vi "Show Animated Busy Icon with Message and Abort Button.vi"(2 "Already active? (F)":bool, 3 "Message":string, 7 "Target VI reference":refnum<vi>, 11 "Error In":errorcluster, 16 "Abort Button Name (Abort)":string="Abort", 17 "Animated Busy Icon Control Name (Animated Busy Icon)":string="Animated Busy Icon", 18 "Message Control Name (Message)":string="Message") -> (10 "Error Out":errorcluster)   [LabVIEW 2021, in "GUI.lvlib"]
doc: "This VI uses error in normally (doesn't do anything if there is an error in) and passes through the error in (ignores additional unternal errors)."
uses:
  GUI/GUI.lvlib
  Utilities/Utilities.lvlib
  Error/Error.lvlib
panel:
  # "see the License on the block diagram (Ctrl+E or Window:Show Block Diagram)"
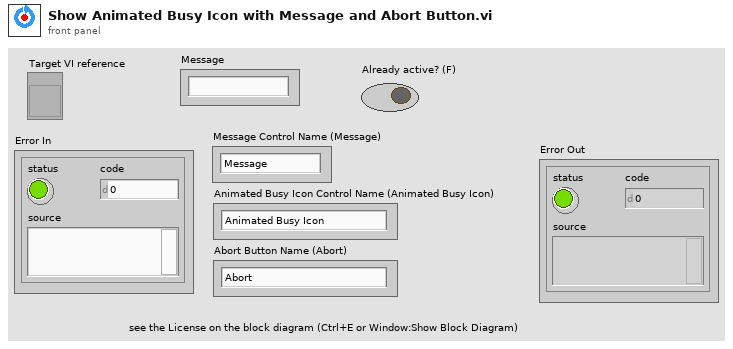
[diagram p1: front panel]
types:
  T1 = enum16{"Controls & Indicators", "Controls", "Indicators"}
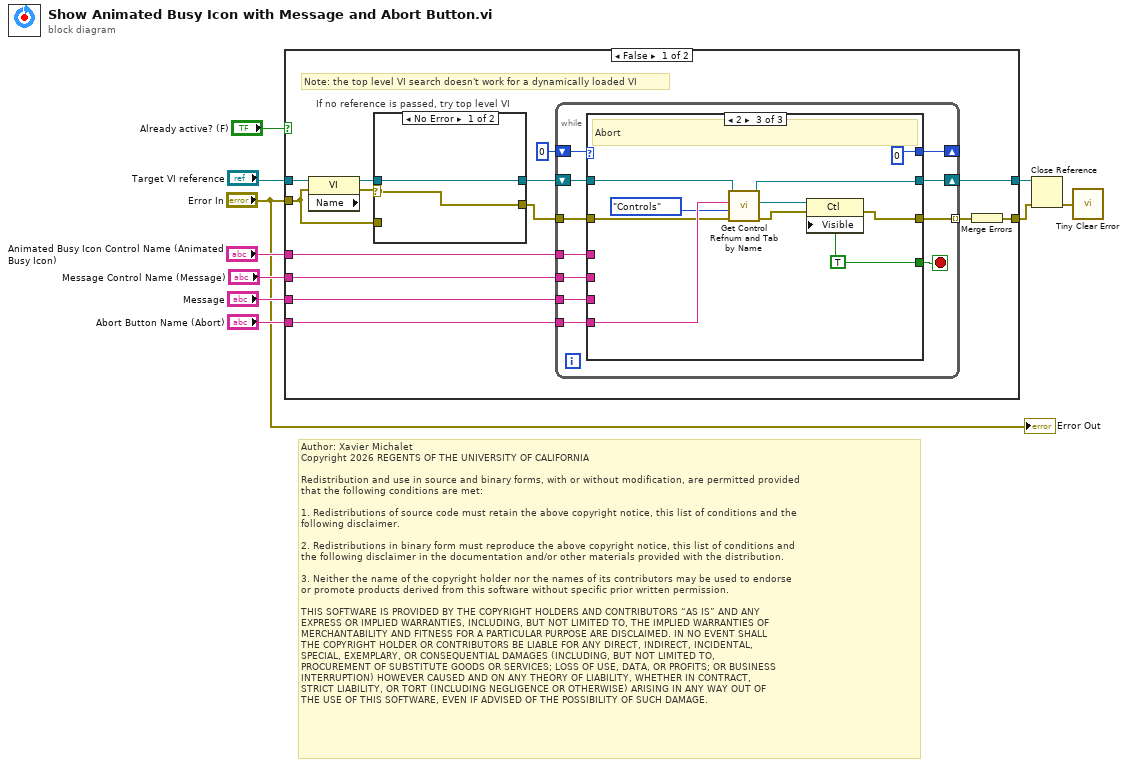
[diagram p0: block diagram]
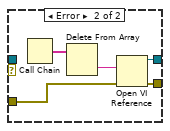
[diagram p2: hidden frame]
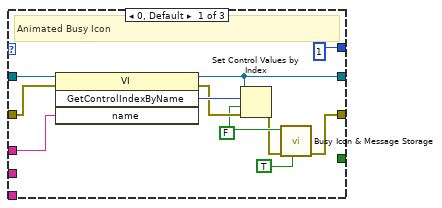
[diagram p3: hidden frame]
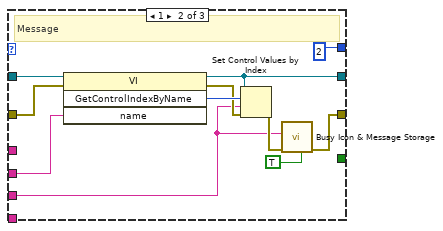
[diagram p4: hidden frame]
diagram:
  # "Author: Xavier Michalet\nCopyright 2026 REGENTS OF THE UNIVERSITY OF CALIFORNIA\n\nRedistribution and use in source and binary forms, with or without modification, are permitted provided\nthat the following conditions are met:\n\n1. Redistributions of source code must retain the above copyright notice, this list of conditions and the\nfollowing disclaimer.\n\n2. Redistributions in binary form must reproduce the above copyright notice, this list of conditions and\nthe following disclaimer in the documentation and/or other materials provided with the distribution.\n\n3. Neither the name of the copyright holder nor the names of its contributors may be used to endorse \nor promote products derived from this software without specific prior written permission.\n\nTHIS SOFTWARE IS PROVIDED BY THE COPYRIGHT HOLDERS AND CONTRIBUTORS “AS IS” AND ANY \nEXPRESS OR IMPLIED WARRANTIES, INCLUDING, BUT NOT LIMITED TO, THE IMPLIED WARRANTIES OF\nMERCHANTABILITY AND FITNESS FOR A PARTICULAR PURPOSE ARE DISCLAIMED. IN NO EVENT SHALL\nTHE COPYRIGHT HOLDER OR CONTRIBUTORS BE LIABLE FOR ANY DIRECT, INDIRECT, INCIDENTAL, \nSPECIAL, EXEMPLARY, OR CONSEQUENTIAL DAMAGES (INCLUDING, BUT NOT LIMITED TO, \nPROCUREMENT OF SUBSTITUTE GOODS OR SERVICES; LOSS OF USE, DATA, OR PROFITS; OR BUSINESS\nINTERRUPTION) HOWEVER CAUSED AND ON ANY THEORY OF LIABILITY, WHETHER IN CONTRACT, \nSTRICT LIABILITY, OR TORT (INCLUDING NEGLIGENCE OR OTHERWISE) ARISING IN ANY WAY OUT OF\nTHE USE OF THIS SOFTWARE, EVEN IF ADVISED OF THE POSSIBILITY OF SUCH DAMAGE."
  n1 = case shown="False" "Already active? (F)" {
    tunnel: [w22 w75] -> w10
    tunnel: [w11 _] -> w9
    tunnel: "Message Control Name (Message)" -> [w19 _]
    tunnel: "Animated Busy Icon Control Name (Animated Busy Icon)" -> [w18 _]
    tunnel: "Message" -> [w17 _]
    tunnel: "Target VI reference" -> [w16 w75]
    tunnel: "Error In" -> [w12 _]
    tunnel: "Abort Button Name (Abort)" -> [w13 _]
    frame False {
      # "Note: the top level VI search doesn't work for a dynamically loaded VI"
      n2 = property class="VI" props=["Name"](reference=w16, error in=w12) -> (reference out=w14:refnum<vi>, error out=w15:errorcluster)  [unwired: 1 out]
      n3 = case "If no reference is passed, try top level VI" shown="No Error" w15 {
        selector: w15 -> [w25 _]
        tunnel: [w25 w31] -> w24
        tunnel: [w26 w30] -> w23
        tunnel: w14 -> [w26 _]
        tunnel: w12 -> [_ w27]
        frame No Error {
        }
        frame Error {
          n4 = Call Chain() -> (call chain=w28:string[])
          n5 = Delete From Array(array=w28) -> (deleted portion=w29:string)  [unwired: 2 in, 1 out]
          n6 = Open VI Reference(vi path=w29, error in (no error)=w27) -> (vi reference=w30:refnum<vi>, error out=w31:errorcluster)  [unwired: 4 in]
        }
      }
      n7 = while {
        shift-right: [w40] -> w22
        shift-left: w23 -> [w41]
        shift-right: [w37] -> _
        shift-left: 0 -> [w38]
        tunnel: w19 -> [w35]
        tunnel: w18 -> [w34]
        tunnel: w17 -> [w33]
        tunnel: w13 -> [w32]
        tunnel: w24 -> [w42]
        tunnel: [w39] -> w21 mode=indexing
        stop <- w36 stop-if-true
        n8 = case shown="2" w38 {
          tunnel: w42 -> [w51 w62 w72]
          tunnel: w41 -> [w50 w61 w70]
          tunnel: [w49 w60 w69] -> w40
          tunnel: [w43 w56 w66] -> w39
          tunnel: [1 2 0] -> w37
          tunnel: [_ _ w65] -> w36
          tunnel: w35 -> [_ w58 _]
          tunnel: w34 -> [w47 _ _]
          tunnel: w33 -> [_ w55 _]
          tunnel: w32 -> [_ _ w73]
          frame 0, Default {
            w46 = FALSE ("Visible")
            # "Animated Busy Icon"
            n9 = invoke class="VI" method="GetControlIndexByName"(reference=w50, error in=w51, "name"=w47) -> (reference out=w49:refnum<vi>, error out=w52:errorcluster, "GetControlIndexByName"=w53:i32)  [unwired: 1 in, 1 out]
            n10 = Set Control Values by Index(0:w49, 1:w53, 2:w46, 3:w52) -> (11:w44:errorcluster)
            n11 = call "Busy Icon & Message Storage.vi"("Get(F)/Set Busy Icon"=TRUE, "Error In"=w44, "Busy Icon Status (F = busy)"=w46) -> ("Error Out"=w43:errorcluster)  [unwired: 6 in, 2 out]
          }
          frame 1 {
            # "Message"
            n12 = invoke class="VI" method="GetControlIndexByName"(reference=w61, error in=w62, "name"=w58) -> (reference out=w60:refnum<vi>, error out=w63:errorcluster, "GetControlIndexByName"=w64:i32)  [unwired: 1 in, 1 out]
            n13 = Set Control Values by Index(0:w60, 1:w64, 2:w55, 3:w63) -> (11:w57:errorcluster)
            n14 = call "Busy Icon & Message Storage.vi"("Get(F)/Set Message"=TRUE, "Error In"=w57, "Message String"=w55) -> ("Error Out"=w56:errorcluster)  [unwired: 6 in, 2 out]
          }
          frame 2 {
            w65 = TRUE
            # "Abort"
            n15 = call "Get Control Refnum and Tab by Name.vi"("error in"=w72, "Selection"=T1."Controls", "Control Label"=w73, "VI  Ref"=w70) -> ("error out"=w67:errorcluster, "Ctl Refnum"=w68:refnum<vi>, "VI  Ref (dup)"=w69:refnum<vi>)  [unwired: 3 in, 2 out]
            n16 = property class="Ctl"(reference=w68, error in=w67, "Visible"=w65) -> (error out=w66:errorcluster)  [unwired: 1 out]
          }
        }
      }
      n17 = Merge Errors(w21) -> (w11:errorcluster)
    }
    frame True {
    }
  }
  n18 = Close Reference(reference=w10, error in (no error)=w9) -> (error out=w1:errorcluster)
  n19 = call "Tiny Clear Error.vi"("Error In"=w1) -> ()  [unwired: 8 in, 1 out]
  "Error Out" <- "Error In"
